vi "ShortestDistanceBetweenRegimesTest.vi"() -> (3 "Were there any errors at all?":bool)   [LabVIEW 2013]
uses:
  Data/TypeDefs/Sailing Regimes.ctl
panel:
  in  "Regime2 inputs":T1[](array[typedef])=[enum."Upwind - Starboard Tack", enum."Tack - Bow across wind", enum."Run - Port Tack", enum."Run - Port Tack", enum."Upwind - Starboard Tack", enum."Reach - Port Tack"]
  out "Are chosen directions right?":bool[](array[boolean])=[TRUE, TRUE, TRUE, TRUE, TRUE, TRUE]
  in  "Expected direction output":i32[](array[numeric])=[1, -1, 0, 1, -1]
  in  "Expected distance output":i32[](array[numeric])=[1, 1, 0, 5, 5]
  out "Actual direction outputs":i32[](array[numeric])
  out "Actual distance outputs":i32[](array[numeric])
  in  "Regime1 inputs":T1[](array[typedef])=[enum."Tack - Bow across wind", enum."Upwind - Starboard Tack", enum."Run - Port Tack", enum."Turn between Upwind/Reach - Starboard Tack", enum."Jibe - Stern across wind", enum."Reach - Port Tack"]
  out "Are chosen distances right?":bool[](array[boolean])=[TRUE, TRUE, TRUE, TRUE, TRUE, TRUE]
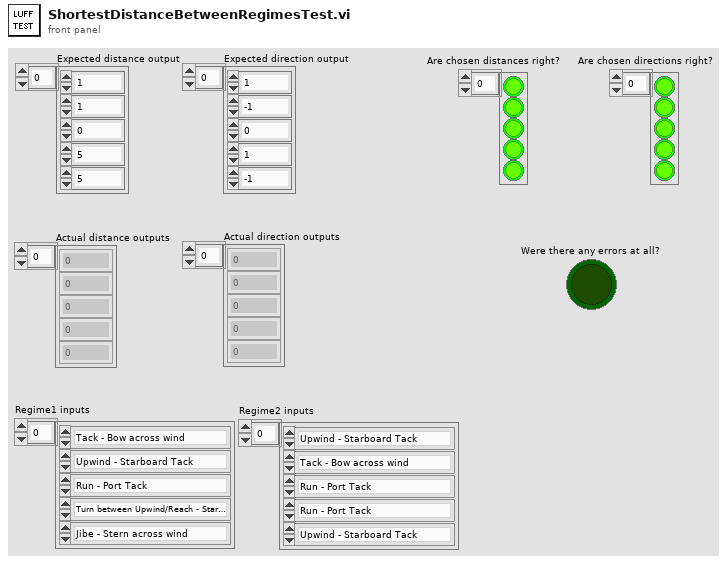
[diagram p1: front panel]
types:
  T1 = typedef "Sailing Regimes.ctl" = enum16{"Tack - Bow across wind", "Upwind - Starboard Tack", "Turn between Upwind/Reach - Starboard Tack", "Reach - Starboard Tack", "Turn between Reach/Run - Starboard Tack", "Run - Starboard Tack", "Jibe - Stern across wind", "Run - Port Tack", "Turn between Reach/Run - Port Tack", "Reach - Port Tack", "Turn between Upwind/Reach - Port Tack", "Upwind - Port Tack"}
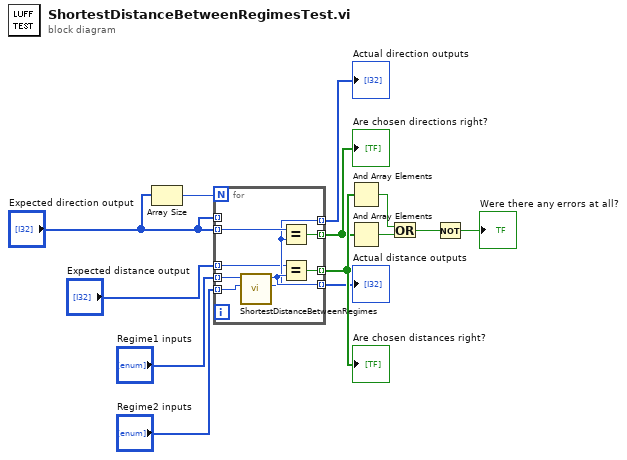
[diagram p0: block diagram]
diagram:
  n1 = Array Size(array="Expected direction output") -> (size(s)=w13:i32)
  n2 = for {
    N: w13 -> [_]
    tunnel: [w21] -> w12 mode=indexing
    tunnel: "Expected direction output" -> [_] mode=indexing
    tunnel: [w20] -> w10 mode=indexing
    tunnel: "Regime1 inputs" -> [w15] mode=indexing
    tunnel: [w18] -> w8 mode=indexing
    tunnel: "Expected distance output" -> [w17] mode=indexing
    tunnel: "Expected direction output" -> [w19] mode=indexing
    tunnel: [w16] -> w3 mode=indexing
    tunnel: "Regime2 inputs" -> [w14] mode=indexing
    n3 = call "ShortestDistanceBetweenRegimes.vi"("Regime 2"=w14, "Regime 1"=w15) -> ("Direction to Regime 2"=w18:i32, "Distance between the two regimes"=w20:i32)  [unwired: 8 in]
    n4 = Equal?(x=w19, y=w18) -> (x = y?=w16:bool)
    n5 = Equal?(x=w17, y=w20) -> (x = y?=w21:bool)
  }
  "Are chosen distances right?" <- w12
  "Actual distance outputs" <- w10
  "Actual direction outputs" <- w8
  "Are chosen directions right?" <- w3
  n6 = And Array Elements(Boolean array=w12) -> (logical AND=w5:bool)
  n7 = And Array Elements(Boolean array=w3) -> (logical AND=w4:bool)
  n8 = Or(x=w5, y=w4) -> (x .or. y?=w6:bool)
  n9 = Not(x=w6) -> (.not. x?=→"Were there any errors at all?":bool)
